vi "Highpass (FPGA).vi"   [LabVIEW 2023]
uses:
  <vilib>/eio/EIONode/EIONode.xnode
  <vilib>/rvi/DataTransferAndStorage/Container/XNode/niFpgaContainer.xnode
  <vilib>/rvi/eio/common/nirviEmuTemplateMethod_errors.vi
  <vilib>/rvi/interface/RandomDataEmulation/nirviRandomDataFpgaReadWriteTemplate.vi
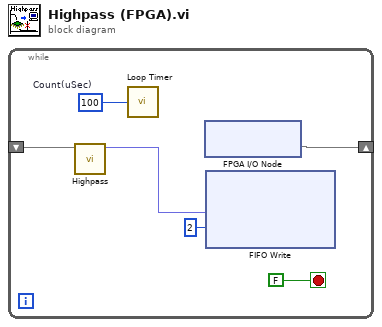
[diagram p0: block diagram]
diagram:
  n1 = while {
    shift-right: [w5] -> _
    shift-left: _ -> [w3]
    stop <- FALSE stop-if-true
    w4 = u16 100  # Count(uSec)
    n2 = call "Highpass.vi"("input data"=w3) -> ("output data"=w2:fxp<+/-,32,7>)  [unwired: 10 out]
    n3 = call "Loop Timer"("Count(uSec)"=w4) -> ()  [unwired: 1 out]
    n4 = xnode "FPGA I/O Node"() -> ("Mod1/AI0"=w5)  [unwired: 1 in, 1 out]
    n5 = xnode ("FIFO Write")("Element"=w2, "Timeout"=2) -> ()  [unwired: 1 in, 2 out]
  }
